vi "IssueCommand-SubVI.vi"(0 "Current Position":dbl, 1 "Max Velocity?":bool, 5 "Calibration":dbl, 7 "Loop Iteration":i32, 9 "Direction":dbl, 11 "ADC/DAC Resolution":i32, 12 "Motion Multiplier":dbl=5.0) -> (4 "Pos. Command":dbl, 8 "Loop Iteration Out":i32)   [LabVIEW 2014]
panel:
  out "dPos":dbl
  # "OUTPUT"
  # "INPUT"
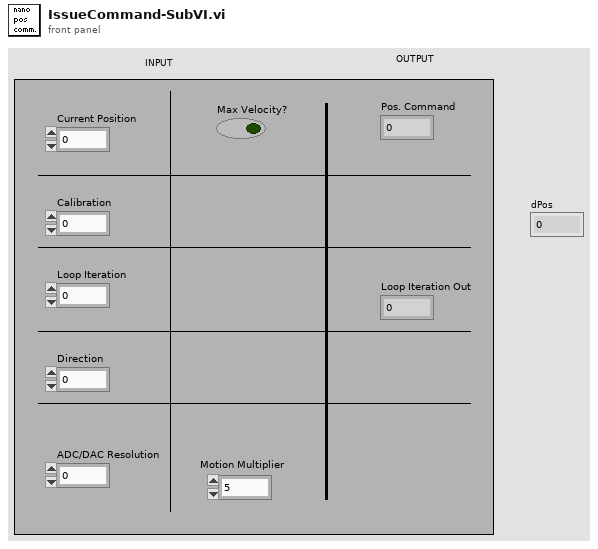
[diagram p1: front panel]
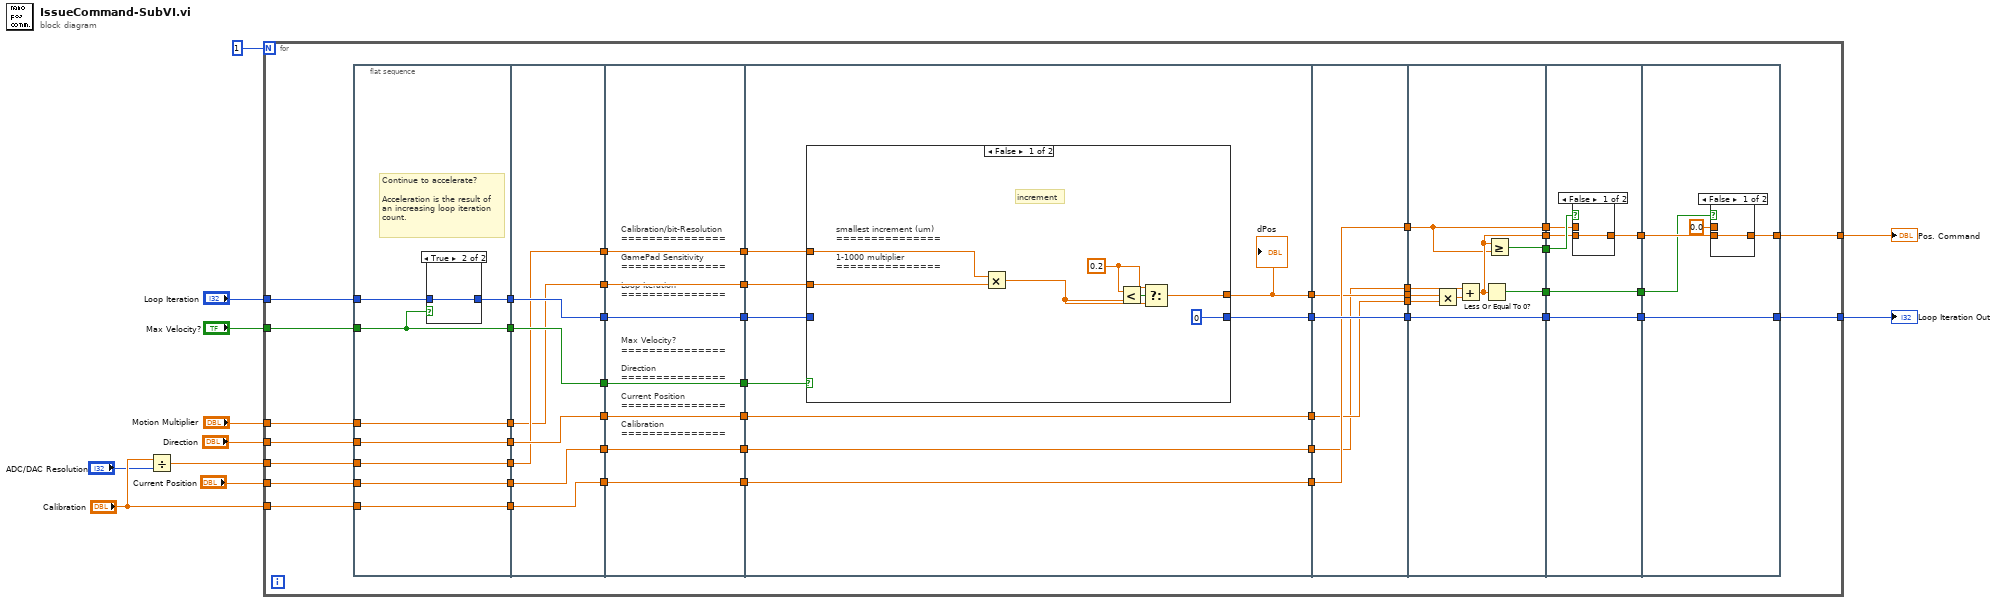
[diagram p0: block diagram]
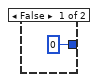
[diagram p2: hidden frame]
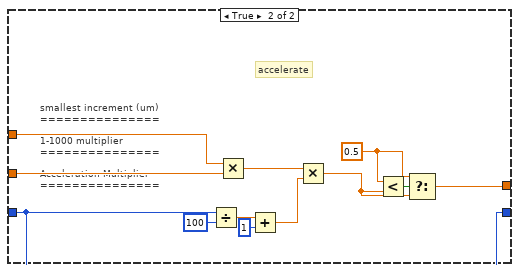
[diagram p3: hidden frame]
diagram:
  n1 = Divide(x="Calibration", y="ADC/DAC Resolution") -> (x/y=w4:dbl)
  n2 = for {
    N: 1 -> [_]
    tunnel: "Calibration" -> [w59]
    tunnel: "Current Position" -> [w54]
    tunnel: "Loop Iteration" -> [w56]
    tunnel: "Direction" -> [w58]
    tunnel: [w57] -> w8
    tunnel: "Max Velocity?" -> [w55]
    tunnel: w4 -> [w53]
    tunnel: "Motion Multiplier" -> [w52]
    tunnel: [w51] -> w2
    n3 = flat-sequence {
      tunnel: w52 -> [w63]
      tunnel: w53 -> [w64]
      tunnel: w54 -> [w65]
      tunnel: w55 -> [w60]
      tunnel: w56 -> [w62]
      tunnel: w58 -> [w66]
      tunnel: w59 -> [w67]
      tunnel: [w67] -> w32
      tunnel: [w66] -> w31
      tunnel: [w61] -> w30
      tunnel: [w60] -> w29
      tunnel: [w65] -> w28
      tunnel: [w64] -> w27
      tunnel: [w63] -> w26
      tunnel: w32 -> [w76]
      tunnel: [w76] -> w25
      tunnel: w31 -> [w75]
      tunnel: [w75] -> w23
      tunnel: w30 -> [w74]
      tunnel: [w74] -> w21
      tunnel: w29 -> [w73]
      tunnel: [w73] -> w19
      tunnel: w28 -> [w72]
      tunnel: [w72] -> w17
      tunnel: w27 -> [w71]
      tunnel: [w71] -> w15
      tunnel: w26 -> [w70]
      tunnel: [w70] -> w13
      tunnel: w25 -> [w83]
      tunnel: [w83] -> w24
      tunnel: w23 -> [w82]
      tunnel: [w82] -> w22
      tunnel: w21 -> [w81]
      tunnel: [w81] -> w20
      tunnel: w19 -> [w80]
      tunnel: [w80] -> w18
      tunnel: w17 -> [w79]
      tunnel: [w79] -> w16
      tunnel: w15 -> [w78]
      tunnel: [w78] -> w14
      tunnel: w13 -> [w77]
      tunnel: [w77] -> w12
      tunnel: [w84] -> w42
      tunnel: [w89] -> w40
      tunnel: [w90] -> w38
      tunnel: [w85] -> w36
      tunnel: [w87] -> w34
      tunnel: w24 -> [w89]
      tunnel: w22 -> [w90]
      tunnel: w20 -> [w88]
      tunnel: w18 -> [w86]
      tunnel: w16 -> [w87]
      tunnel: w14 -> [w92]
      tunnel: w12 -> [w91]
      tunnel: w42 -> [w116]
      tunnel: [w116] -> w41
      tunnel: w40 -> [w115]
      tunnel: [w115] -> w39
      tunnel: w38 -> [w114]
      tunnel: [w114] -> w37
      tunnel: w36 -> [w113]
      tunnel: [w113] -> w35
      tunnel: w34 -> [w112]
      tunnel: [w112] -> w33
      tunnel: [w123] -> w47
      tunnel: w41 -> [w125]
      tunnel: [w125] -> w46
      tunnel: [w122] -> w45
      tunnel: [w118] -> w44
      tunnel: w39 -> [w117]
      tunnel: [w117] -> w43
      tunnel: w37 -> [w121]
      tunnel: w35 -> [w120]
      tunnel: w33 -> [w119]
      tunnel: w47 -> [w128]
      tunnel: [w126] -> w50
      tunnel: w46 -> [w131]
      tunnel: [w131] -> w49
      tunnel: [w130] -> w48
      tunnel: w45 -> [w130]
      tunnel: w44 -> [w129]
      tunnel: w43 -> [w127]
      tunnel: [w138] -> w51
      tunnel: [w135] -> w57
      tunnel: w50 -> [w136]
      tunnel: w49 -> [w138]
      tunnel: w48 -> [w134]
      frame #0 {
        # "Continue to accelerate?\n\nAcceleration is the result of\nan increasing loop iteration\ncount."
        n4 = case shown="True" w60 {
          tunnel: [0 ("Loop Iteration") w69] -> w61
          tunnel: w62 -> [_ w69]
          frame False {
          }
          frame True {
          }
        }
      }
      frame #1 {
      }
      frame #2 {
        # "Calibration/bit-Resolution\n===============\n\nGamePad Sensitivity\n===============\n\nLoop Iteration\n===============\n\n\n\n\nMax Velocity?\n===============\n\nDirection\n===============\n\nCurrent Position\n===============\n\nCalibration\n==============="
      }
      frame #3 {
        n5 = case shown="False" w86 {
          tunnel: [w98 w110] -> w85
          tunnel: w88 -> [_ w101]
          tunnel: [0 ("Loop Iteration") w101] -> w84
          tunnel: w91 -> [w96 w108]
          tunnel: w92 -> [w95 w107]
          frame False {
            w97 = 0.2
            # "smallest increment (um)\n===============\n\n1-1000 multiplier\n==============="
            # "increment"
            n6 = Multiply(x=w95, y=w96) -> (x*y=w94:dbl)
            n7 = Less?(x=w97, y=w94) -> (x < y?=w99:bool)
            n8 = Select(t=w97, s=w99, f=w94) -> (s? t:f=w98:dbl)
          }
          frame True {
            w109 = 0.5
            # "smallest increment (um)\n===============\n\n1-1000 multiplier\n===============\n\nAcceleration Multiplier\n==============="
            # "accelerate"
            n9 = Divide(x=w101, y=100) -> (x/y=w103:dbl)
            n10 = Multiply(x=w107, y=w108) -> (x*y=w106:dbl)
            n11 = Add(x=w103, y=1) -> (x+y=w100:dbl)
            n12 = Multiply(x=w106, y=w100) -> (x*y=w102:dbl)
            n13 = Less?(x=w109, y=w102) -> (x < y?=w111:bool)
            n14 = Select(t=w109, s=w111, f=w102) -> (s? t:f=w110:dbl)
          }
        }
        "dPos" <- w85
      }
      frame #4 {
      }
      frame #5 {
        n15 = Multiply(x=w120, y=w121) -> (x*y=w124:dbl)
        n16 = Add(x=w119, y=w124) -> (x+y=w123:dbl)
        n17 = Less Or Equal To 0?(x=w123) -> (x <= 0?=w122:bool)
        n18 = Greater Or Equal?(x=w123, y=w117) -> (x >= y?=w118:bool)
      }
      frame #6 {
        n19 = case shown="False" w129 {
          tunnel: w127 -> [_ w133]
          tunnel: [w132 w133] -> w126
          tunnel: w128 -> [w132 _]
          frame False {
          }
          frame True {
          }
        }
      }
      frame #7 {
        n20 = case shown="False" w134 {
          tunnel: 0.0 ("Calibration") -> [_ w140]
          tunnel: [w139 w140] -> w135
          tunnel: w136 -> [w139 _]
          frame False {
          }
          frame True {
          }
        }
      }
    }
  }
  "Pos. Command" <- w8
  "Loop Iteration Out" <- w2
